vi "Adapt Class To Cluster.vi"() -> ()   [LabVIEW 2016]
doc: "This VI demonstrates a function of the GCraftsman JSON Serialization Toolkit.\n\nIt uses the 'Adapt to Type' function to convert a LabVIEW Object to a cluster datatype. It performs best-fit matching, handling out-of-order and missing or extra items. \nIt also successfully adapts nested objects or hierarchical class data.\n\nThis does not require the class to have accessor methods"
uses:
  ExampleCluster.ctl
  Class2/Class2.lvclass
  C:/GCraftsman/Products/JSON Toolkit/JSON Object Serialization/Example/Class1/Class1.lvclass
  Class3/Class3.lvclass
  JSON Object Serialization/GCraftsman JSON Serialization/GCraftsman JSON Serialization.lvlib
panel:
  in  "myBool":bool=TRUE
  in  "anotherNumber":dbl=123.0 format="%#_13g"
  in  "someNumber":dbl=456.0 format="%#_13g"
  in  "myNum 2":dbl=555.0 format="%#_13g"
  in  "myNum":dbl=444.0 format="%#_13g"
  out "Cluster":T1
  # "This VI demonstrates a function of the GCraftsman JSON Serialization Toolkit.\n\nLook at the block diagram to see that the 'Adapt to Type' function can convert a LabVIEW Object to a cluster datatype.   It performs best-fit match, handling out-of-order and missing or extra items.  \nIt also successfully adapts nested objects or hierarchical class data.\n\nThis does not require the class to have accessor methods"
  # "Object Data"
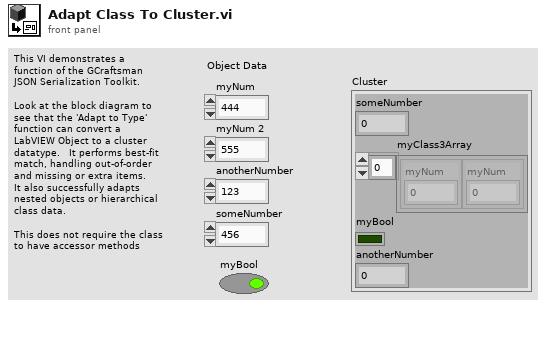
[diagram p1: front panel]
types:
  T1 = typedef "ExampleCluster.ctl" = cluster{"someNumber":dbl, "myClass3Array":cluster{"myNum":dbl}[], "myBool":bool, "anotherNumber":dbl}
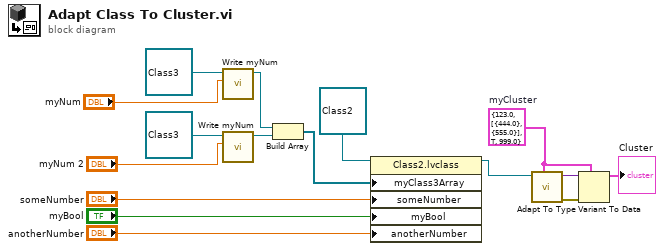
[diagram p0: block diagram]
diagram:
  w14 = T1 {"someNumber"=123.0, "myClass3Array"=[{"myNum"=444.0}, {"myNum"=555.0}], "myBool"=TRUE, "anotherNumber"=999.0}  # myCluster
  n1 = call-dynamic "Write myNum.vi"("myNum"="myNum", "Test3 in"=refnum<class "Class3.lvclass"> refnum ("Test3.lvclass")) -> ("Test3 out"=w7:refnum<class "Class3.lvclass">)  [unwired: 8 in, 1 out]
  n2 = call-dynamic "Write myNum.vi"("myNum"="myNum 2", "Test3 in"=refnum<class "Class3.lvclass"> refnum ("Test3.lvclass")) -> ("Test3 out"=w10:refnum<class "Class3.lvclass">)  [unwired: 8 in, 1 out]
  n3 = Build Array(w7, w10) -> (w5:refnum<class "Class3.lvclass">[])
  n4 = property class="Class2.lvclass"(reference=refnum<class "Class2.lvclass"> refnum ("Test2.lvclass"), "myClass3Array"=w5, "someNumber"="someNumber", "myBool"="myBool", "anotherNumber"="anotherNumber") -> (reference out=w1:refnum<class "Class2.lvclass">)  [unwired: 1 in, 1 out]
  n5 = call "Adapt To Type.vi"("Type and Defaults"=w14, "Variant in"=w1) -> ("error out"=w16:errorcluster, "Variant out"=w15:variant)  [unwired: 8 in]
  n6 = Variant To Data(error in=w16, type=w14, Variant=w15) -> (data=→"Cluster":T1)  [unwired: 1 out]
